vi "Tegam4040 - Calibration.vi"(0 "Instrument Session Handle In":u32 format="%x", 1 "Calibration":T1(ring), 11 "error in (no error)":errorcluster) -> (4 "Instrument Session Handle Out (dupl)":u32 format="%x", 15 "error out":errorcluster)   [LabVIEW 2010, in "Tegam4040.lvlib"]
doc: "Calibration: This bit selects mode of input coupling.\n\n0: Disable Calibration (default)\n1: Enable Calibration\n\nIf Calibration is enabled it will disable Attenuation bits."
uses:
  Tegam4040.lvlib
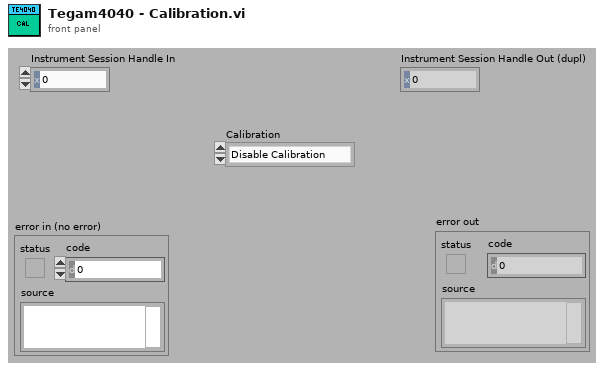
[diagram p1: front panel]
types:
  T1 = enum16{"Disable Calibration", "Enable Calibration"}
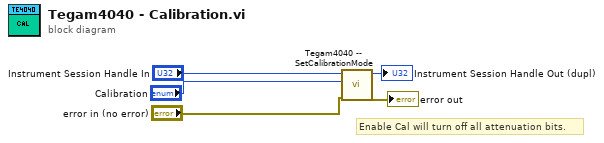
[diagram p0: block diagram]
diagram:
  # "Enable Cal will turn off all attenuation bits."
  n1 = call "Tegam4040 -- SetCalibrationMode.vi"("error in (no error)"="error in (no error)", "Calibration"="Calibration", "Instrument Session Handle In"="Instrument Session Handle In") -> ("error out"=→"error out":errorcluster, "Instrument Session Handle Out (dupl)"=→"Instrument Session Handle Out (dupl)":u32)  [unwired: 7 in]
